vi "triger.vi"(9 "frequene echantillonage":i32, 10 "Signal":waveform(dbl) caption="waveform") -> (2 "waveform en sortie":waveform(dbl))   [LabVIEW 2013]
panel:
  out "indice fractionnaire ou x":dbl
  out "Y":dbl[](array[numeric])
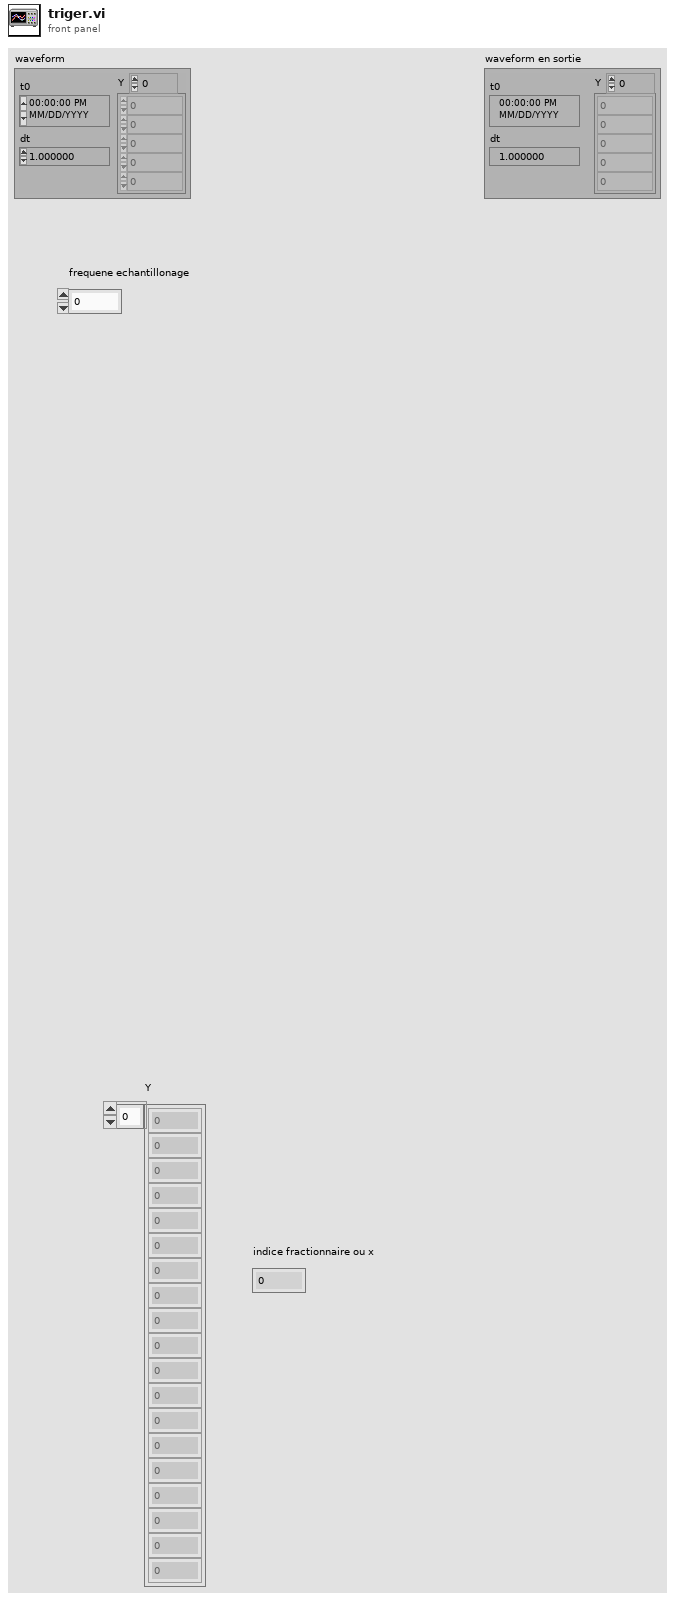
[diagram p1: front panel]
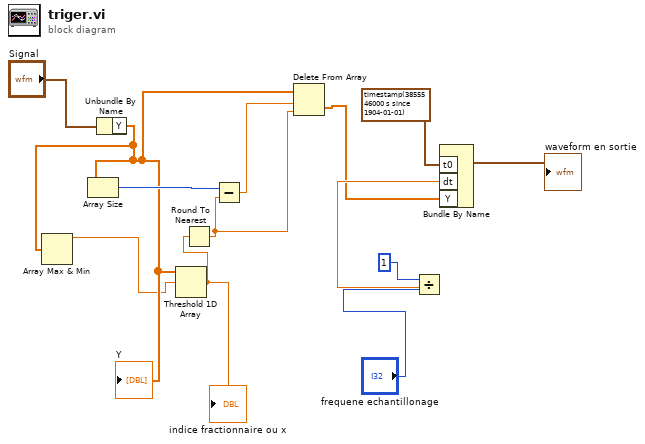
[diagram p0: block diagram]
diagram:
  n1 = Unbundle By Name("Signal") -> ("Y"=w5:dbl[])
  "Y" <- w5
  n2 = Array Max & Min(array=w5) -> (max value=w4:dbl)  [unwired: 3 out]
  n3 = Array Size(array=w5) -> (size(s)=w13:i32)
  n4 = Threshold 1D Array(2:w4, 3:w5) -> (0:w8:dbl)  [unwired: 1 in]
  "indice fractionnaire ou x" <- w8
  n5 = Round To Nearest(number=w8) -> (nearest integer value=w7:dbl)
  n6 = Subtract(x=w13, y=w7) -> (x-y=w6:dbl)
  n7 = Delete From Array(array=w5, length=w6, index=w7) -> (deleted portion=w3:dbl[])  [unwired: 1 out]
  n8 = Divide(x=1, y="frequene echantillonage") -> (x/y=w11:dbl)
  n9 = Bundle By Name("t0"=timestamp(3855546000 s since 1904-01-01), "dt"=w11, "Y"=w3) -> (→"waveform en sortie":waveform(dbl))  [unwired: 1 in]
